vi "Download REV 2m Distance Sensor Driver.vi"() -> ()   [LabVIEW 2020]
uses:
  <vilib>/nisyscfg/Close (System).vi
  <vilib>/WebDAVClient/NI_WebDAV.lvlib
  <vilib>/nisyscfg/nisyscfg.lvlib
panel:
  out "String":string="Downloading REV 2m Distance Sensor Driver to roboRIO"
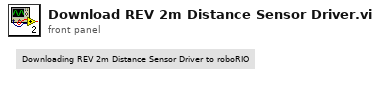
[diagram p1: front panel]
types:
  T1 = typedef "NI_WebDAV.lvlib/SessionHandle.ctl" = refnum<k1>
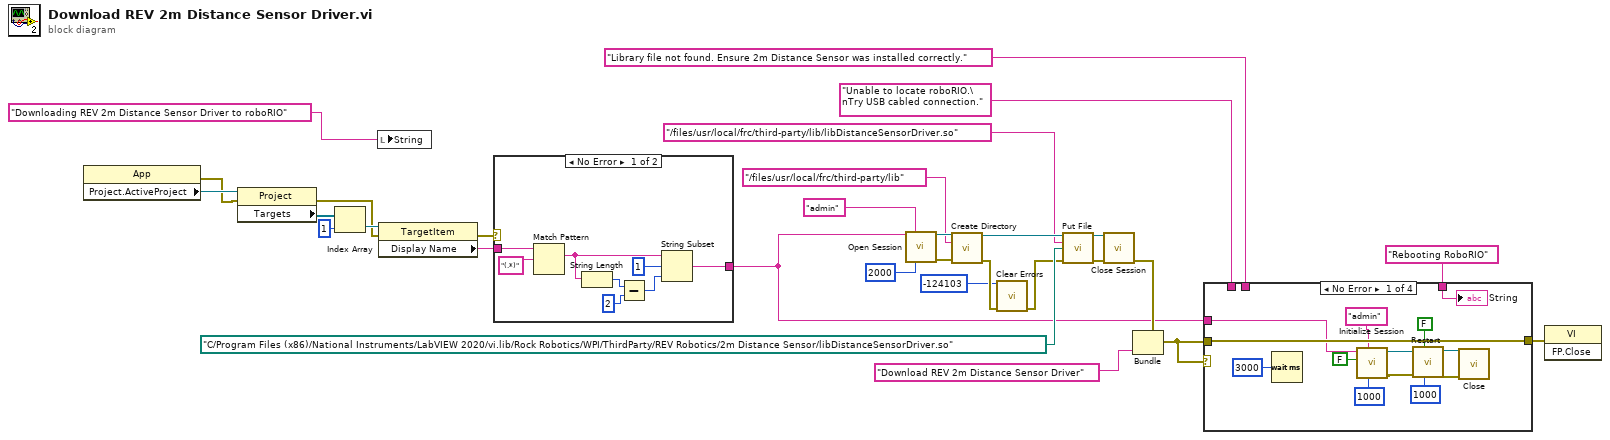
[diagram p0: block diagram]
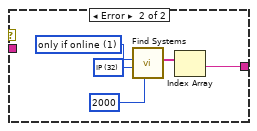
[diagram p2: hidden frame]
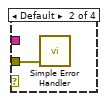
[diagram p3: hidden frame]
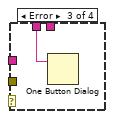
[diagram p4: hidden frame]
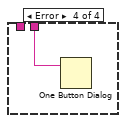
[diagram p5: hidden frame]
diagram:
  n1 = property class="App"() -> (error out=w17:errorcluster, "Project.ActiveProject"=w30:refnum<vi>)  [unwired: 2 in, 1 out]
  n2 = property class="Project"(reference=w30, error in=w17) -> (error out=w16:errorcluster, "Targets"=w29:refnum<vi>[])  [unwired: 1 out]
  n3 = Index Array(array=w29, index=1) -> (element=w28:refnum<vi>)
  n4 = local write "String"("Downloading REV 2m Distance Sensor Driver to roboRIO" ("String")) -> ()
  n5 = property class="TargetItem"(reference=w28, error in=w16) -> (error out=w4:errorcluster, "Display Name"=w12:string)  [unwired: 1 out]
  n6 = case shown="No Error" w4 {
    tunnel: w12 -> [w32 _]
    tunnel: [w31 w40] -> w3
    frame No Error {
      n7 = Match Pattern(string=w32, regular expression="(.*)") -> (match substring=w36:string)  [unwired: 1 in, 3 out]
      n8 = String Length(string=w36) -> (length=w35:i32)
      n9 = Subtract(x=w35, y=2 ("offset (0)")) -> (x-y=w33:i32)
      n10 = String Subset(string=w36, offset (0)=1, length (rest)=w33) -> (substring=w31:string)
    }
    frame Error {
      w39 = u32 32 items=["Hostname"=16, "Hostname (IP)"=18, "Hostname (MAC)"=19, "IP"=32, "IP (Hostname)"=33, "IP (MAC)"=35, "MAC"=48, "MAC (Hostname)"=49, "MAC (IP)"=50] ("Output (Hostname and IP)")
      w43 = u32 1 items=["none"=0, "only if online"=1, "all"=3] ("Include Cached Results (all)")
      n11 = call <vilib>:"Find Systems.vi"("Timeout (4000 ms)"=u32 2000, "Output (Hostname and IP)"=w39, "Include Cached Results (all)"=w43) -> ("Detected Systems"=w41:string[])  [unwired: 6 in, 2 out]
      n12 = Index Array(array=w41) -> (element=w40:string)  [unwired: 1 in]
    }
  }
  n13 = call <vilib>:"Open Session.vi"("host uri prefix"=w3, "username"="admin", "timeout ms"=2000) -> ("session handle out"=w26:T1, "error out"=w25:errorcluster)  [unwired: 11 in]
  n14 = call <vilib>:"Create Directory.vi"("session handle"=w26, "relative uri"="/files/usr/local/frc/third-party/lib" ("file uri"), "error in (no error)"=w25) -> ("session handle out"=w23:T1, "error out"=w11:errorcluster)  [unwired: 11 in]
  n15 = call <vilib>:"Clear Errors.vi"("error in (no error)"=w11, "specific error code to clear (0: all)"=-124103) -> ("error out"=w9:errorcluster)  [unwired: 4 in, 1 out]
  n16 = call <vilib>:"Put File.vi"("session handle"=w23, "relative uri"="/files/usr/local/frc/third-party/lib/libDistanceSensorDriver.so" ("file uri"), "local file path"=path "C:/Program Files (x86)/National Instruments/LabVIEW 2020/vi.lib/Rock Robotics/WPI/ThirdParty/REV Robotics/2m Distance Sensor/libDistanceSensorDriver.so", "error in (no error)"=w9) -> ("session handle out"=w22:T1, "error out"=w24:errorcluster)  [unwired: 9 in, 1 out]
  n17 = call <vilib>:"Close Session.vi"("session handle"=w22, "error in (no error)"=w24) -> ("error out"=w15:errorcluster)  [unwired: 13 in]
  n18 = Bundle(cluster=w15, "source"="Download REV 2m Distance Sensor Driver" ("error source (\" \")")) -> (w14:errorcluster)  [unwired: 2 in]
  n19 = case shown="No Error" w14 {
    tunnel: w14 -> [w54 w57 _ _]
    tunnel: "Unable to locate roboRIO.\nTry USB cabled connection." ("message") -> [_ _ w58 _]
    tunnel: "Rebooting RoboRIO" ("message") -> [w56 _ _ _]
    tunnel: [w54 _ _ _] -> w6
    tunnel: w3 -> [w45 _ _ _]
    tunnel: "Library file not found. Ensure 2m Distance Sensor was installed correctly." ("message") -> [_ _ _ w59]
    frame No Error {
      n20 = Wait (ms)(milliseconds to wait=u32 3000) -> ()  [unwired: 1 out]
      n21 = call <vilib>:"Initialize Session.vi"("Connect Timeout (4000 ms)"=u32 1000, "User Name"="admin" ("username"), "Force Property Refresh (T)"=FALSE, "Target (localhost)"=w45) -> ("error out"=w50:errorcluster, "Session out"=w53:refnum<k21>)  [unwired: 6 in]
      n22 = call <vilib>:"Restart.vi"("Timeout (180,000 ms)"=u32 1000, "Wait Until Complete (T)"=FALSE, "error in (no error)"=w50, "Session in"=w53) -> ("error out"=w51:errorcluster, "Session out"=w52:refnum<k21>)  [unwired: 5 in, 1 out]
      n23 = call-poly <vilib>:"Close.vi"("error in (no error)"=w51, "Session in"=w52) -> ()  [unwired: 9 in, 1 out]
      "String" <- w56
    }
    frame Default {
      n24 = call <vilib>:"Simple Error Handler.vi"("error in (no error)"=w57) -> ()  [unwired: 4 in, 5 out]
    }
    frame Error {
      n25 = One Button Dialog(message=w58) -> ()  [unwired: 1 in, 1 out]
    }
    frame Error {
      n26 = One Button Dialog(message=w59) -> ()  [unwired: 1 in, 1 out]
    }
  }
  n27 = invoke class="VI" method="FP.Close"(error in=w6) -> ()  [unwired: 2 in, 3 out]
